vi "LFA_Initialize.vi"(8 "error in (no error)":errorcluster, 10 "Is Visible?":bool=TRUE) -> (0 "error out":errorcluster, 3 "LightField Automation out":refnum<class "LightField Automation.lvclass">)   [LabVIEW 2019, in "LightField Automation.lvclass"]
uses:
  LightField Automation.lvclass
  C:/Program Files/Princeton Instruments/LightField/AddInViews/PrincetonInstruments.LightFieldViewV3.dll
  C:/Program Files/Princeton Instruments/LightField/PrincetonInstruments.LightField.AutomationV3.dll
  LightField Automation.lvclass/LightField Automation.ctl
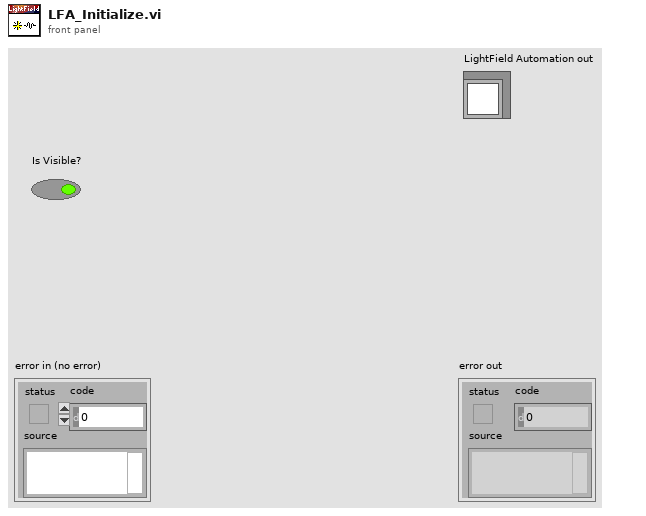
[diagram p1: front panel]
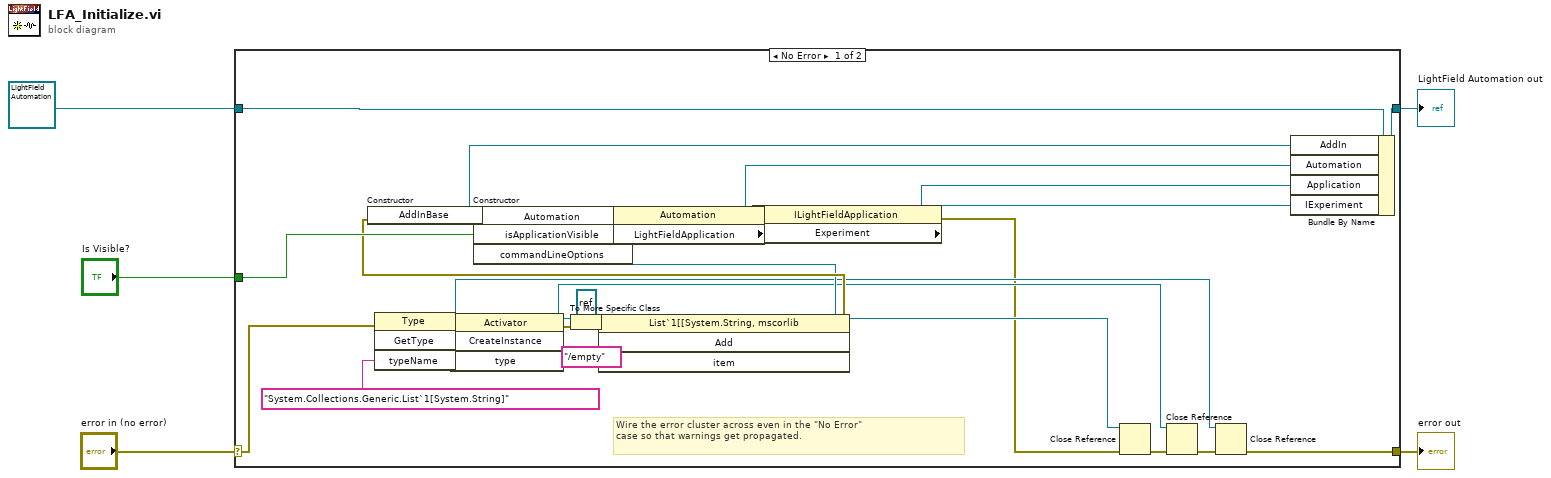
[diagram p0: block diagram]
diagram:
  n1 = case shown="No Error" "error in (no error)" {
    selector: "error in (no error)" -> [w22 w37]
    tunnel: [w12 w37] -> w4
    tunnel: [w35 w36] -> w3
    tunnel: refnum<class "LightField Automation.lvclass"> refnum ("LightField Automation.lvclass") -> [w24 w36]
    tunnel: "Is Visible?" -> [w32 _]
    frame No Error {
      # "Wire the error cluster across even in the \"No Error\"\ncase so that warnings get propagated."
      n2 = invoke class="Type" method="GetType"(error in=w22, "typeName"="System.Collections.Generic.List`1[System.String]") -> (reference out=w7:refnum<k24>, error out=w20:errorcluster, "GetType"=w21:refnum<k24>)  [unwired: 2 in, 1 out]
      n3 = invoke class="Activator" method="CreateInstance"(error in=w20, "type"=w21) -> (reference out=w8:refnum<k24>, error out=w19:errorcluster, "CreateInstance"=w18:refnum<k24>)  [unwired: 2 in, 1 out]
      n4 = To More Specific Class(target class=refnum<k24> refnum ("commandLineOptions"), reference=w18, error in=w19) -> (specific class reference=w16:refnum<k24>, error out=w15:errorcluster)
      n5 = invoke class="List`1[[System.String, mscorlib" method="Add"(reference=w16, error in=w15, "item"="/empty") -> (reference out=w9:refnum<k24>, error out=w13:errorcluster)  [unwired: 1 in, 2 out]
      n6 = constructor class="AddInBase"(error in=w13) -> (reference out=w31:refnum<k24>, error out=w30:errorcluster)  [unwired: 2 in, 1 out]
      n7 = constructor class="Automation"(error in=w30, "isApplicationVisible"=w32, "commandLineOptions"=w9) -> (reference out=w29:refnum<k24>, error out=w28:errorcluster)  [unwired: 2 in, 3 out]
      n8 = property class="Automation"(reference=w29, error in=w28) -> (reference out=w27:refnum<k24>, error out=w25:errorcluster, "LightFieldApplication"=w26:refnum<k24>)
      n9 = property class="ILightFieldApplication"(reference=w26, error in=w25) -> (reference out=w33:refnum<k24>, error out=w6:errorcluster, "Experiment"=w34:refnum<k24>)
      n10 = Close Reference(reference=w9, error in (no error)=w6) -> (error out=w10:errorcluster)
      n11 = Close Reference(reference=w8, error in (no error)=w10) -> (error out=w11:errorcluster)
      n12 = Close Reference(reference=w7, error in (no error)=w11) -> (error out=w12:errorcluster)
      n13 = Bundle By Name(cluster=w24, "AddIn"=w31, "Automation"=w27, "Application"=w33, "IExperiment"=w34) -> (w35:refnum<class "LightField Automation.lvclass">)
    }
    frame Error {
    }
  }
  "error out" <- w4
  "LightField Automation out" <- w3
